vi "Disconnect.vi"(8 "error in (no error)":errorcluster, 11 "Picomoto8742ControllerClass in":refnum<class "Picomoto8742ControllerClass.lvclass">) -> (0 "error out":errorcluster, 3 "Picomoto8742ControllerClass out":refnum<class "Picomoto8742ControllerClass.lvclass">)   [LabVIEW 2013, in "Picomoto8742ControllerClass.lvclass"]
doc: "Disconnect from the physical device"
uses:
  Picomoto8742ControllerClass.lvclass
  Picomoto8742ControllerClass.lvclass/Picomoto8742ControllerClass.ctl
  PicoMotor8472Comm/PicoMotor8742Comm.lvclass
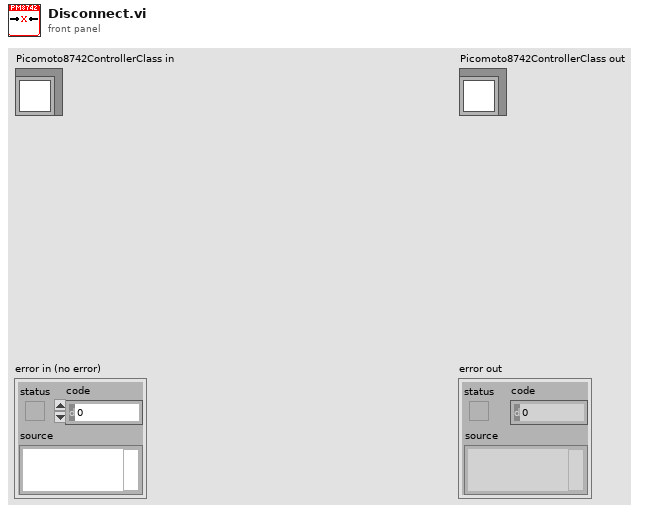
[diagram p1: front panel]
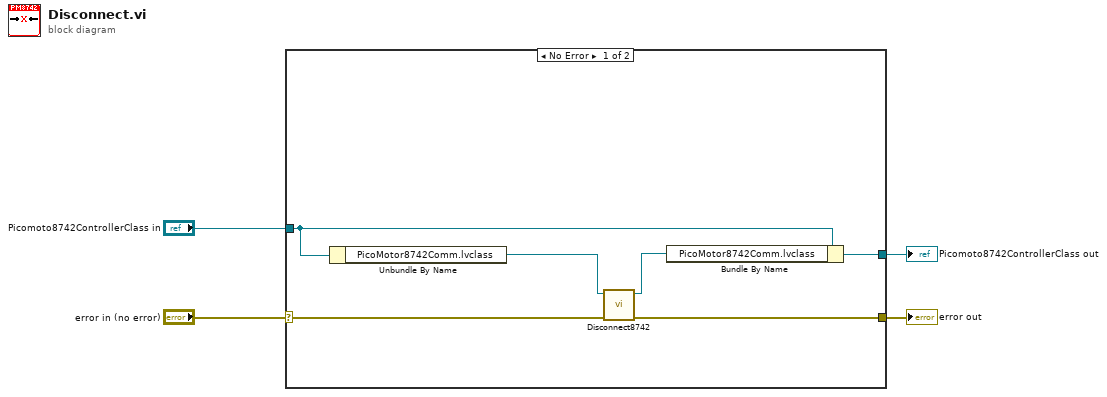
[diagram p0: block diagram]
diagram:
  n1 = case shown="No Error" "error in (no error)" {
    selector: "error in (no error)" -> [w10 w12]
    tunnel: [w9 w12] -> w3
    tunnel: [w5 w11] -> w1
    tunnel: "Picomoto8742ControllerClass in" -> [w6 w11]
    frame No Error {
      n2 = Unbundle By Name(w6) -> ("PicoMotor8742Comm.lvclass"=w8:refnum<class "PicoMotor8742Comm.lvclass">)
      n3 = call-dynamic "Disconnect8742.vi"("error in (no error)"=w10, "Picomotor8742Comm in"=w8) -> ("error out"=w9:errorcluster, "Picomotor8742Comm out"=w7:refnum<class "PicoMotor8742Comm.lvclass">)  [unwired: 8 in]
      n4 = Bundle By Name(cluster=w6, "PicoMotor8742Comm.lvclass"=w7) -> (w5:refnum<class "Picomoto8742ControllerClass.lvclass">)
    }
    frame Error {
    }
  }
  "error out" <- w3
  "Picomoto8742ControllerClass out" <- w1
